vi "NumIntegrate_Rkdp_Func_B1.vi"(11 "Index":i32) -> (3 "RKDP_B1":dbl)   [LabVIEW 2019, in "Trajectory_Library.lvlib"]
doc: "Internal function used by Rkdp_Impl.vi\n\nInputs:\n - Index -- Index into B1 array (must be 0 - 6 )\n\nOutputs:\n - B1 -- Value looked up by index."
uses:
  Trajectory_Library.lvlib
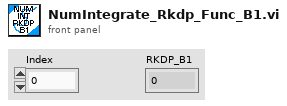
[diagram p1: front panel]
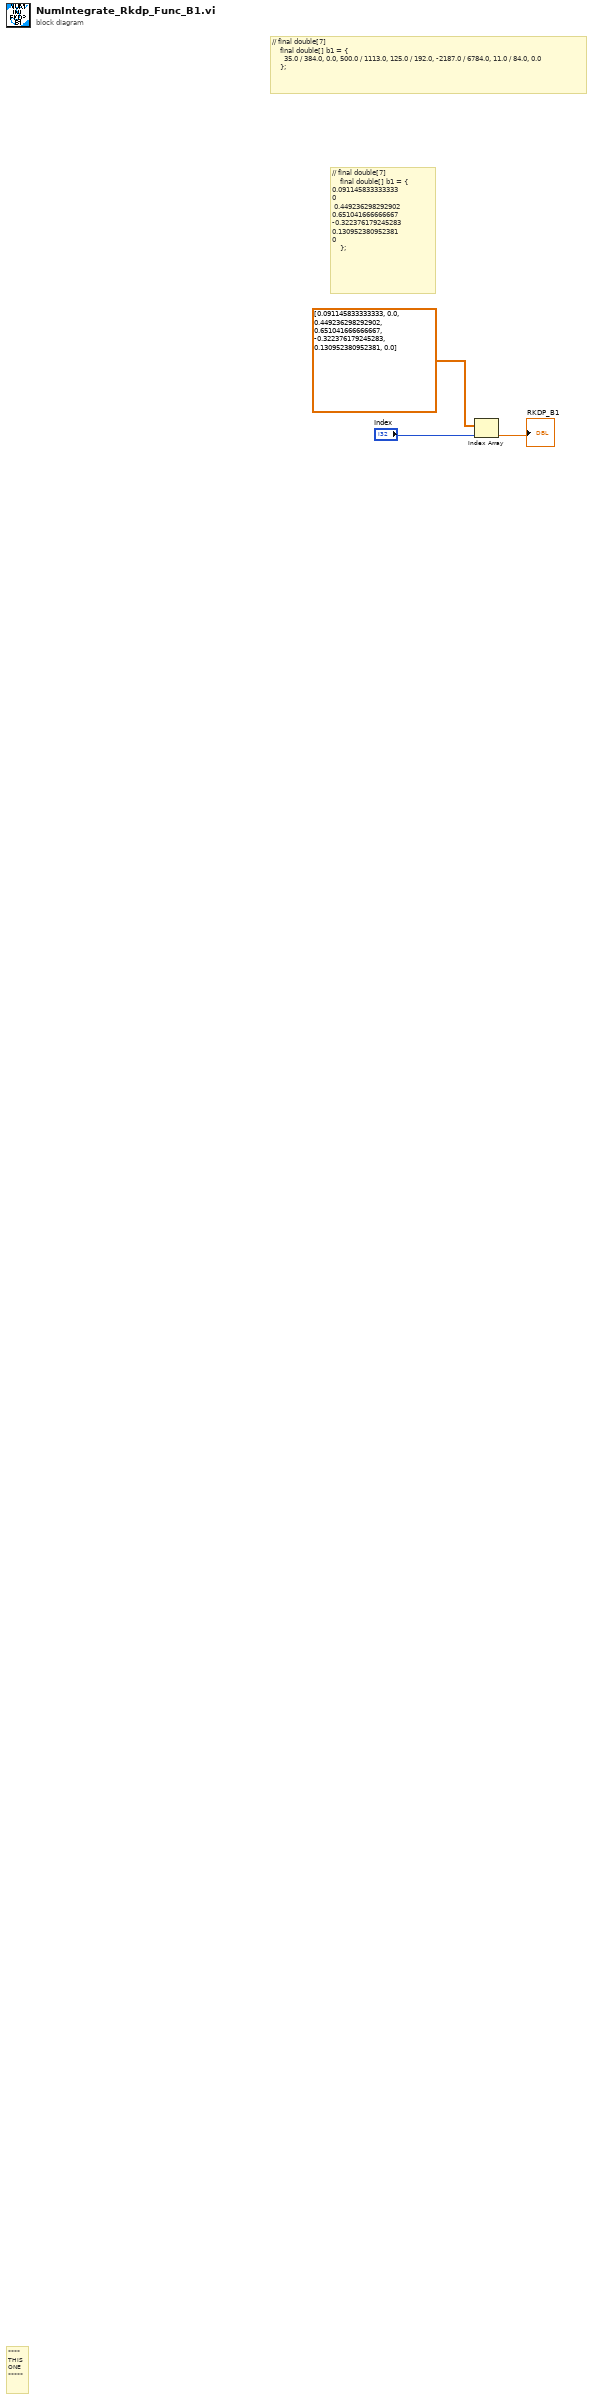
[diagram p0: block diagram]
diagram:
  # "// final double[7]\t\t\t\t\t\t\n    final double[] b1 = {\t\t\t\t\t\t\n0.091145833333333\t    \n0\t   \n 0.449236298292902\t    \n0.651041666666667\t    \n-0.322376179245283\t    \n0.130952380952381\t\n0\n    };"
  # "// final double[7]\n    final double[] b1 = {\n      35.0 / 384.0, 0.0, 500.0 / 1113.0, 125.0 / 192.0, -2187.0 / 6784.0, 11.0 / 84.0, 0.0\n    };"
  # "****\nTHIS\nONE\n*****"
  n1 = Index Array(array=dbl[] [0.091145833333333, 0.0, 0.449236298292902, 0.651041666666667, -0.322376179245283, 0.130952380952381, 0.0], index="Index") -> (element=→"RKDP_B1":dbl)
